vi "test_1.vi"() -> ()   [LabVIEW 2014]
panel:
  in  "VALVE  64":bool
  in  "VALVE  63":bool
  in  "VALVE  62":bool
  in  "VALVE  61":bool
  in  "VALVE  60":bool
  in  "VALVE  59":bool
  in  "VALVE  58":bool
  in  "VALVE  57":bool
  in  "VALVE  56":bool
  in  "VALVE  55":bool
  in  "VALVE  54":bool
  in  "VALVE  53":bool
  in  "VALVE  52":bool
  in  "VALVE  51":bool
  in  "VALVE  50":bool
  in  "VALVE  49":bool
  in  "VALVE  48":bool
  in  "VALVE  47":bool
  in  "VALVE  46":bool
  in  "VALVE  45":bool
  in  "VALVE  44":bool
  in  "VALVE  43":bool
  in  "VALVE  42":bool
  in  "VALVE  41":bool
  in  "VALVE  40":bool
  in  "VALVE  39":bool
  in  "VALVE  38":bool
  in  "VALVE  37":bool
  in  "VALVE  36":bool
  in  "VALVE  35":bool
  in  "VALVE  34":bool
  in  "VALVE  33":bool
  in  "VALVE  32":bool
  in  "VALVE  31":bool
  in  "VALVE  30":bool
  in  "VALVE  29":bool
  in  "VALVE  28":bool
  in  "VALVE  27":bool
  in  "VALVE  26":bool
  in  "VALVE  25":bool
  in  "VALVE  24":bool
  in  "VALVE  23":bool
  in  "VALVE  22":bool
  in  "VALVE  21":bool
  in  "VALVE  20":bool
  in  "VALVE  19":bool
  in  "VALVE  18":bool
  in  "VALVE  17":bool
  in  "VALVE 16":bool
  in  "VALVE  15":bool
  in  "VALVE  14":bool
  in  "VALVE  13":bool
  in  "VALVE  12":bool
  in  "VALVE  11":bool
  in  "VALVE  10":bool
  in  "VALVE  9":bool
  in  "VALVE  8":bool
  in  "VALVE  7":bool
  in  "VALVE  6":bool
  in  "VALVE  5":bool
  in  "VALVE  4":bool
  in  "VALVE  3":bool
  in  "VALVE  2":bool
  in  "VALVE 1":bool
  # "AIR JET\n                    MANUAL CONTROLS"
  # "SLOT 1 DIGITAL OUTPUT CONTROL"
  # "SLOT 2 DIGITAL OUTPUT CONTROL"
  # "DESIGNED BY BOMET TEAM"
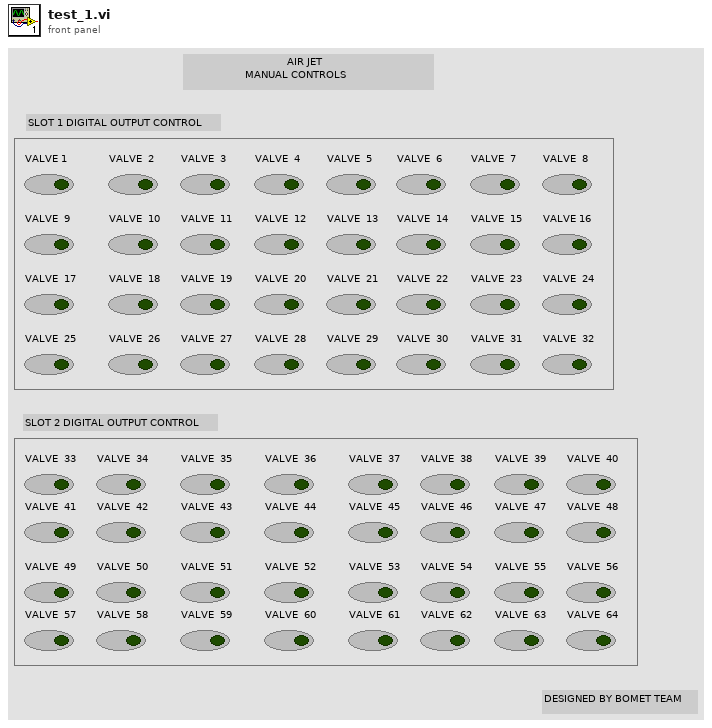
[diagram p1: front panel]
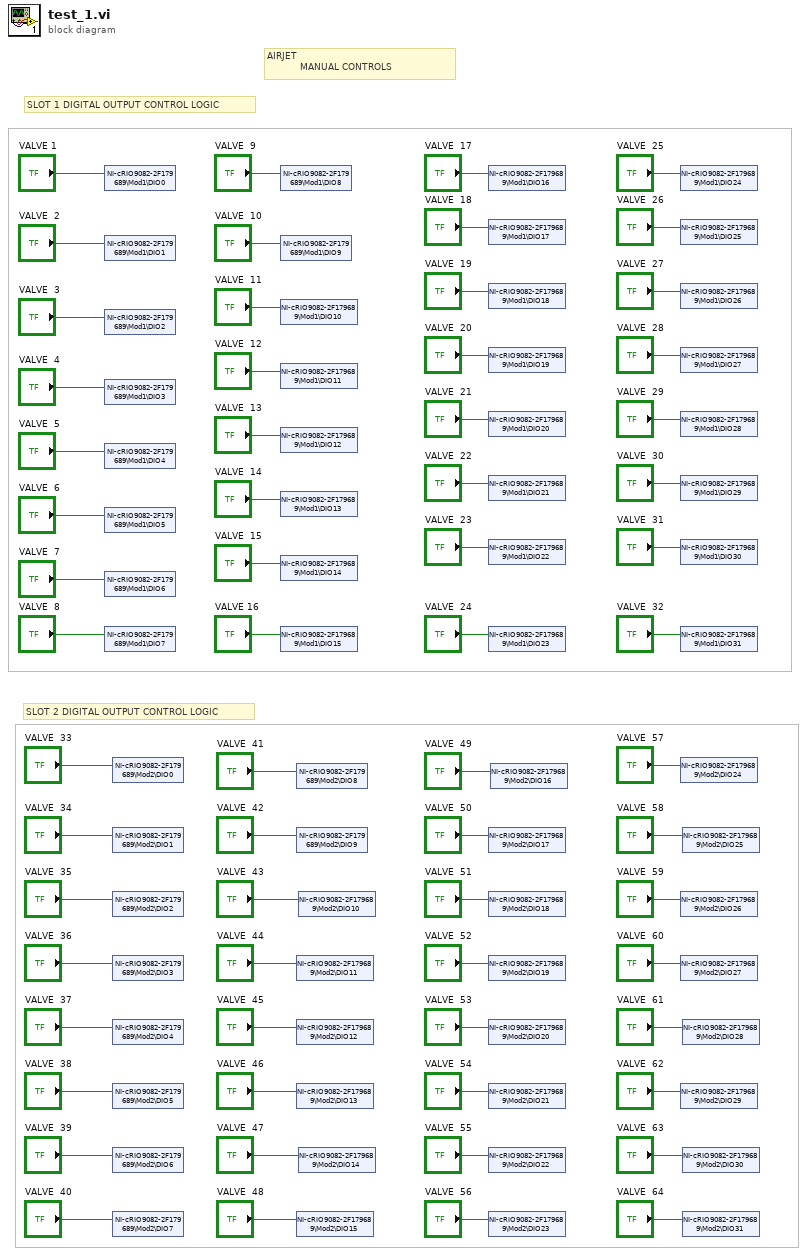
[diagram p0: block diagram]
diagram:
  # "AIRJET\n           MANUAL CONTROLS"
  # "SLOT 2 DIGITAL OUTPUT CONTROL LOGIC"
  # "SLOT 1 DIGITAL OUTPUT CONTROL LOGIC"
  n1 = shared-variable "NI-cRIO9082-2F179689\\Mod1\\DIO0"("VALVE 1") -> ()  [unwired: 1 in, 1 out]
  n2 = shared-variable "NI-cRIO9082-2F179689\\Mod1\\DIO1"("VALVE  2") -> ()  [unwired: 1 in, 1 out]
  n3 = shared-variable "NI-cRIO9082-2F179689\\Mod1\\DIO2"("VALVE  3") -> ()  [unwired: 1 in, 1 out]
  n4 = shared-variable "NI-cRIO9082-2F179689\\Mod1\\DIO3"("VALVE  4") -> ()  [unwired: 1 in, 1 out]
  n5 = shared-variable "NI-cRIO9082-2F179689\\Mod1\\DIO4"("VALVE  5") -> ()  [unwired: 1 in, 1 out]
  n6 = shared-variable "NI-cRIO9082-2F179689\\Mod1\\DIO5"("VALVE  6") -> ()  [unwired: 1 in, 1 out]
  n7 = shared-variable "NI-cRIO9082-2F179689\\Mod1\\DIO6"("VALVE  7") -> ()  [unwired: 1 in, 1 out]
  n8 = shared-variable "NI-cRIO9082-2F179689\\Mod1\\DIO7"("VALVE  8") -> ()  [unwired: 1 in, 1 out]
  n9 = shared-variable "NI-cRIO9082-2F179689\\Mod2\\DIO0"("VALVE  33") -> ()  [unwired: 1 in, 1 out]
  n10 = shared-variable "NI-cRIO9082-2F179689\\Mod2\\DIO1"("VALVE  34") -> ()  [unwired: 1 in, 1 out]
  n11 = shared-variable "NI-cRIO9082-2F179689\\Mod2\\DIO2"("VALVE  35") -> ()  [unwired: 1 in, 1 out]
  n12 = shared-variable "NI-cRIO9082-2F179689\\Mod2\\DIO3"("VALVE  36") -> ()  [unwired: 1 in, 1 out]
  n13 = shared-variable "NI-cRIO9082-2F179689\\Mod2\\DIO4"("VALVE  37") -> ()  [unwired: 1 in, 1 out]
  n14 = shared-variable "NI-cRIO9082-2F179689\\Mod2\\DIO5"("VALVE  38") -> ()  [unwired: 1 in, 1 out]
  n15 = shared-variable "NI-cRIO9082-2F179689\\Mod2\\DIO6"("VALVE  39") -> ()  [unwired: 1 in, 1 out]
  n16 = shared-variable "NI-cRIO9082-2F179689\\Mod2\\DIO7"("VALVE  40") -> ()  [unwired: 1 in, 1 out]
  n17 = shared-variable "NI-cRIO9082-2F179689\\Mod1\\DIO8"("VALVE  9") -> ()  [unwired: 1 in, 1 out]
  n18 = shared-variable "NI-cRIO9082-2F179689\\Mod1\\DIO9"("VALVE  10") -> ()  [unwired: 1 in, 1 out]
  n19 = shared-variable "NI-cRIO9082-2F179689\\Mod1\\DIO10"("VALVE  11") -> ()  [unwired: 1 in, 1 out]
  n20 = shared-variable "NI-cRIO9082-2F179689\\Mod1\\DIO11"("VALVE  12") -> ()  [unwired: 1 in, 1 out]
  n21 = shared-variable "NI-cRIO9082-2F179689\\Mod1\\DIO12"("VALVE  13") -> ()  [unwired: 1 in, 1 out]
  n22 = shared-variable "NI-cRIO9082-2F179689\\Mod1\\DIO13"("VALVE  14") -> ()  [unwired: 1 in, 1 out]
  n23 = shared-variable "NI-cRIO9082-2F179689\\Mod1\\DIO14"("VALVE  15") -> ()  [unwired: 1 in, 1 out]
  n24 = shared-variable "NI-cRIO9082-2F179689\\Mod1\\DIO15"("VALVE 16") -> ()  [unwired: 1 in, 1 out]
  n25 = shared-variable "NI-cRIO9082-2F179689\\Mod2\\DIO8"("VALVE  41") -> ()  [unwired: 1 in, 1 out]
  n26 = shared-variable "NI-cRIO9082-2F179689\\Mod2\\DIO9"("VALVE  42") -> ()  [unwired: 1 in, 1 out]
  n27 = shared-variable "NI-cRIO9082-2F179689\\Mod2\\DIO11"("VALVE  44") -> ()  [unwired: 1 in, 1 out]
  n28 = shared-variable "NI-cRIO9082-2F179689\\Mod2\\DIO12"("VALVE  45") -> ()  [unwired: 1 in, 1 out]
  n29 = shared-variable "NI-cRIO9082-2F179689\\Mod2\\DIO13"("VALVE  46") -> ()  [unwired: 1 in, 1 out]
  n30 = shared-variable "NI-cRIO9082-2F179689\\Mod2\\DIO15"("VALVE  48") -> ()  [unwired: 1 in, 1 out]
  n31 = shared-variable "NI-cRIO9082-2F179689\\Mod2\\DIO10"("VALVE  43") -> ()  [unwired: 1 in, 1 out]
  n32 = shared-variable "NI-cRIO9082-2F179689\\Mod2\\DIO14"("VALVE  47") -> ()  [unwired: 1 in, 1 out]
  n33 = shared-variable "NI-cRIO9082-2F179689\\Mod1\\DIO16"("VALVE  17") -> ()  [unwired: 1 in, 1 out]
  n34 = shared-variable "NI-cRIO9082-2F179689\\Mod1\\DIO17"("VALVE  18") -> ()  [unwired: 1 in, 1 out]
  n35 = shared-variable "NI-cRIO9082-2F179689\\Mod1\\DIO18"("VALVE  19") -> ()  [unwired: 1 in, 1 out]
  n36 = shared-variable "NI-cRIO9082-2F179689\\Mod1\\DIO19"("VALVE  20") -> ()  [unwired: 1 in, 1 out]
  n37 = shared-variable "NI-cRIO9082-2F179689\\Mod1\\DIO20"("VALVE  21") -> ()  [unwired: 1 in, 1 out]
  n38 = shared-variable "NI-cRIO9082-2F179689\\Mod1\\DIO21"("VALVE  22") -> ()  [unwired: 1 in, 1 out]
  n39 = shared-variable "NI-cRIO9082-2F179689\\Mod1\\DIO22"("VALVE  23") -> ()  [unwired: 1 in, 1 out]
  n40 = shared-variable "NI-cRIO9082-2F179689\\Mod1\\DIO23"("VALVE  24") -> ()  [unwired: 1 in, 1 out]
  n41 = shared-variable "NI-cRIO9082-2F179689\\Mod2\\DIO17"("VALVE  50") -> ()  [unwired: 1 in, 1 out]
  n42 = shared-variable "NI-cRIO9082-2F179689\\Mod2\\DIO18"("VALVE  51") -> ()  [unwired: 1 in, 1 out]
  n43 = shared-variable "NI-cRIO9082-2F179689\\Mod2\\DIO19"("VALVE  52") -> ()  [unwired: 1 in, 1 out]
  n44 = shared-variable "NI-cRIO9082-2F179689\\Mod2\\DIO20"("VALVE  53") -> ()  [unwired: 1 in, 1 out]
  n45 = shared-variable "NI-cRIO9082-2F179689\\Mod2\\DIO21"("VALVE  54") -> ()  [unwired: 1 in, 1 out]
  n46 = shared-variable "NI-cRIO9082-2F179689\\Mod2\\DIO22"("VALVE  55") -> ()  [unwired: 1 in, 1 out]
  n47 = shared-variable "NI-cRIO9082-2F179689\\Mod2\\DIO23"("VALVE  56") -> ()  [unwired: 1 in, 1 out]
  n48 = shared-variable "NI-cRIO9082-2F179689\\Mod2\\DIO16"("VALVE  49") -> ()  [unwired: 1 in, 1 out]
  n49 = shared-variable "NI-cRIO9082-2F179689\\Mod1\\DIO24"("VALVE  25") -> ()  [unwired: 1 in, 1 out]
  n50 = shared-variable "NI-cRIO9082-2F179689\\Mod1\\DIO25"("VALVE  26") -> ()  [unwired: 1 in, 1 out]
  n51 = shared-variable "NI-cRIO9082-2F179689\\Mod1\\DIO26"("VALVE  27") -> ()  [unwired: 1 in, 1 out]
  n52 = shared-variable "NI-cRIO9082-2F179689\\Mod1\\DIO27"("VALVE  28") -> ()  [unwired: 1 in, 1 out]
  n53 = shared-variable "NI-cRIO9082-2F179689\\Mod1\\DIO28"("VALVE  29") -> ()  [unwired: 1 in, 1 out]
  n54 = shared-variable "NI-cRIO9082-2F179689\\Mod1\\DIO29"("VALVE  30") -> ()  [unwired: 1 in, 1 out]
  n55 = shared-variable "NI-cRIO9082-2F179689\\Mod1\\DIO30"("VALVE  31") -> ()  [unwired: 1 in, 1 out]
  n56 = shared-variable "NI-cRIO9082-2F179689\\Mod1\\DIO31"("VALVE  32") -> ()  [unwired: 1 in, 1 out]
  n57 = shared-variable "NI-cRIO9082-2F179689\\Mod2\\DIO24"("VALVE  57") -> ()  [unwired: 1 in, 1 out]
  n58 = shared-variable "NI-cRIO9082-2F179689\\Mod2\\DIO26"("VALVE  59") -> ()  [unwired: 1 in, 1 out]
  n59 = shared-variable "NI-cRIO9082-2F179689\\Mod2\\DIO27"("VALVE  60") -> ()  [unwired: 1 in, 1 out]
  n60 = shared-variable "NI-cRIO9082-2F179689\\Mod2\\DIO29"("VALVE  62") -> ()  [unwired: 1 in, 1 out]
  n61 = shared-variable "NI-cRIO9082-2F179689\\Mod2\\DIO25"("VALVE  58") -> ()  [unwired: 1 in, 1 out]
  n62 = shared-variable "NI-cRIO9082-2F179689\\Mod2\\DIO28"("VALVE  61") -> ()  [unwired: 1 in, 1 out]
  n63 = shared-variable "NI-cRIO9082-2F179689\\Mod2\\DIO30"("VALVE  63") -> ()  [unwired: 1 in, 1 out]
  n64 = shared-variable "NI-cRIO9082-2F179689\\Mod2\\DIO31"("VALVE  64") -> ()  [unwired: 1 in, 1 out]
